vi "find_angles_3d.vi"(9 "Vect 2":cluster{"X":dbl, "Y":dbl, "Z":dbl}, 10 "Vect 1":cluster{"X":dbl, "Y":dbl, "Z":dbl}) -> (2 "angle":dbl)   [LabVIEW 2020, in "3DPC_SurfacePlot.xctl"]
uses:
  <vilib>/Native 3D Graph/xcontrol/3DPC_SurfacePlot.xctl
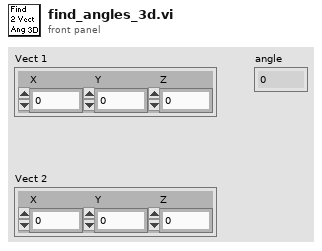
[diagram p1: front panel]
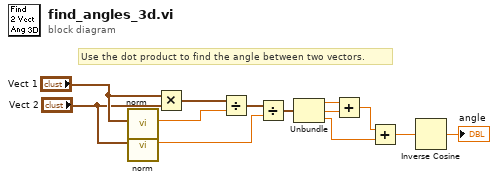
[diagram p0: block diagram]
diagram:
  # "Use the dot product to find the angle between two vectors."
  n1 = call <vilib>:"norm.vi"("Vector"="Vect 1") -> ("Norm"=w7:sgl)  [unwired: 10 out]
  n2 = call <vilib>:"norm.vi"("Vector"="Vect 2") -> ("Norm"=w6:sgl)  [unwired: 10 out]
  n3 = Multiply(x="Vect 1", y="Vect 2") -> (x*y=w11:cluster{"X":dbl, "Y":dbl, "Z":dbl})
  n4 = Divide(x=w11, y=w7) -> (x/y=w10:cluster{"X":dbl, "Y":dbl, "Z":dbl})
  n5 = Divide(x=w10, y=w6) -> (x/y=w9:cluster{"X":dbl, "Y":dbl, "Z":dbl})
  n6 = Unbundle(w9) -> ("X"=w5:dbl, "Y"=w4:dbl, "Z"=w3:dbl)
  n7 = Add(x=w5, y=w4) -> (x+y=w2:dbl)
  n8 = Add(x=w2, y=w3) -> (x+y=w1:dbl)
  n9 = Inverse Cosine(1:w1) -> (0:→"angle":dbl)
